vi "averager.vi"() -> ()   [LabVIEW 2015]
uses:
  <vilib>/Utility/file.llb/Write Delimited Spreadsheet (DBL).vi
  <vilib>/imath/engines/lvmath2/RunTimeEngine/Managers/WorkSpace/UID Generator.vi
  <vilib>/imath/engines/lvmath2/RunTimeEngine/BuiltInFunctions/length/NIMS_length(GV).vi
  <instcachedir>/0/NIMS_length(GV)_08A3D13377FD4E4B96F5795FBF3698FA.lvgen/NIMS_length(GV)_08A3D13377FD4E4B96F5795FBF3698FA_000.vi
  <vilib>/imath/engines/lvmath2/RunTimeEngine/RangeToken/NIMS_Range_R2 - Integer.vi
  <instcachedir>/0/NIMS_Range_R2 - Integer_396D5D4FB869421F9245109A0975AD54.lvgen/NIMS_Range_R2 - Integer_396D5D4FB869421F9245109A0975AD54_000.vi
  <vilib>/imath/engines/lvmath2/RunTimeEngine/CommandStatement/MC_CommandStatement_break.vi
  <vilib>/imath/engines/lvmath2/RunTimeEngine/VariableToken/NIMS_VariableToken_CondDefinedDefinedByReplace.vi
  <instcachedir>/0/NIMS_VariableToken_CondDefinedDefinedByReplace_D162CFFC24174562A9FEA619A91E1A56.lvgen/NIMS_VariableToken_CondDefinedDefinedByReplace_D162CFFC24174562A9FEA619A91E1A56_002.vi
  <vilib>/imath/engines/lvmath2/RunTimeEngine/IndexRead/NIMS V(S).vi
  <instcachedir>/0/NIMS V(S)_0488751826AF41519A22953C041130DC.lvgen/NIMS V(S)_0488751826AF41519A22953C041130DC_000.vi
  <vilib>/imath/engines/lvmath2/RunTimeEngine/IndexReplace/NIMS V(S)=S.vi
  <instcachedir>/0/NIMS V(S)=S_9916D32195284AEB9D40BA9A64F3B0C5.lvgen/NIMS V(S)=S_9916D32195284AEB9D40BA9A64F3B0C5_000.vi
  <vilib>/imath/engines/lvmath2/RunTimeEngine/RunTimeType/NIMS_RunTimeType_From StrictType (excl LVString).vi
  <instcachedir>/0/NIMS_RunTimeType_From StrictType (excl LVString)_EB1C38A9BC5048DA9ABDA8F781E54D21.lvgen/NIMS_RunTimeType_From StrictType (excl LVString)_EB1C38A9BC5048DA9ABDA8F781E54D21_000.vi
  <vilib>/imath/engines/lvmath2/RunTimeEngine/ErrorHandling/NIMS_Create Error From Enums.vi
  <vilib>/imath/engines/lvmath2/RunTimeEngine/LocalVariableDefStatement/MC_LocalVariableDefStatement_Display.vi
  <vilib>/imath/engines/lvmath2/RunTimeEngine/VariableToken/NIMS_VariableToken_CondDefined.vi
  <instcachedir>/0/NIMS_VariableToken_CondDefined_FE30D0A1BFB24F098D41DEBABFE96BE1.lvgen/NIMS_VariableToken_CondDefined_FE30D0A1BFB24F098D41DEBABFE96BE1_003.vi
  <vilib>/imath/engines/lvmath2/RunTimeEngine/BuiltInFunctions/sum/NIMS_sum(GV).vi
  <instcachedir>/0/NIMS_sum(GV)_67F5EC36BC034E54A6BEC5B0673C00E5.lvgen/NIMS_sum(GV)_67F5EC36BC034E54A6BEC5B0673C00E5_000.vi
  <vilib>/imath/engines/lvmath2/RunTimeEngine/Managers/SymbolTable/Clear UID.vi
  <vilib>/imath/engines/lvmath2/RunTimeEngine/NodeEndStatement/NIMS_NodeEndStatement_Output.vi
  <instcachedir>/0/NIMS_NodeEndStatement_Output_53EC0D466D134D7ABD903AC30B43404B.lvgen/NIMS_NodeEndStatement_Output_53EC0D466D134D7ABD903AC30B43404B_001.vi
  <vilib>/imath/engines/lvmath2/RunTimeEngine/ErrorHandling/NIMS_Finalize Error.vi
  <vilib>/imath/engines/lvmath2/RunTimeEngine/Managers/SymbolTable/NIMS_WorkSpace.lvlib
panel:
  in  "R2":dbl
  out "Average Resistance":dbl
  in  "Path":path
  out "data 5":dbl
  out "data 4":dbl
  out "data 3":dbl
  out "data 2":dbl
  out "data":dbl
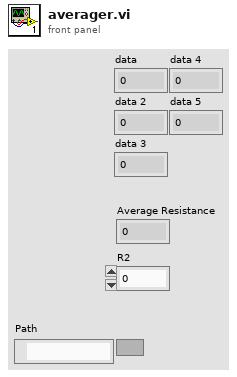
[diagram p1: front panel]
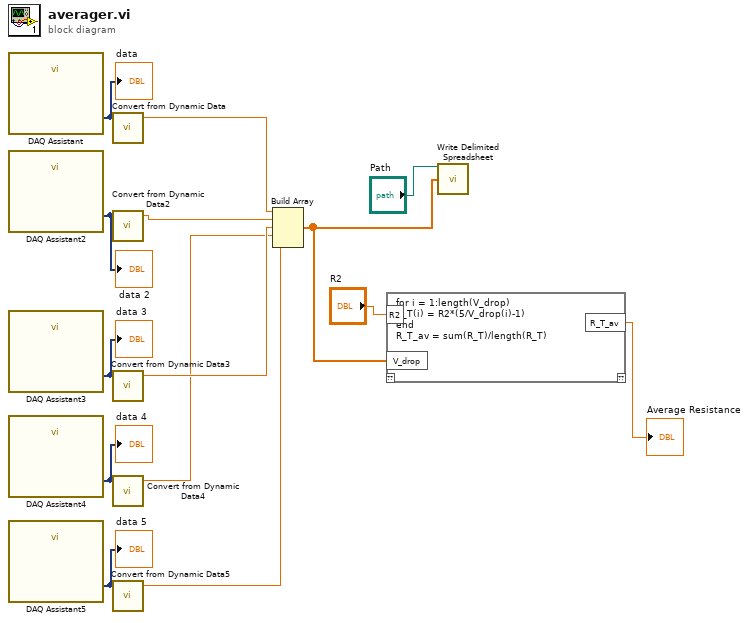
[diagram p0: block diagram]
diagram:
  n1 = call "DAQ Assistant"() -> ("data"=w14:dynamicdata)  [unwired: 17 in, 2 out]
  "data" <- w14
  n2 = call "DAQ Assistant2"() -> ("data"=w10:dynamicdata)  [unwired: 17 in, 2 out]
  "data 2" <- w10
  n3 = call "DAQ Assistant3"() -> ("data"=w11:dynamicdata)  [unwired: 17 in, 2 out]
  "data 3" <- w11
  n4 = call "DAQ Assistant4"() -> ("data"=w12:dynamicdata)  [unwired: 17 in, 2 out]
  "data 4" <- w12
  n5 = call "DAQ Assistant5"() -> ("data"=w13:dynamicdata)  [unwired: 17 in, 2 out]
  "data 5" <- w13
  n6 = call "Convert from Dynamic Data"("Dynamic Data Type"=w14) -> ("Scalar"=w9:dbl)  [unwired: 3 in]
  n7 = call "Convert from Dynamic Data2"("Dynamic Data Type"=w10) -> ("Scalar"=w8:dbl)  [unwired: 3 in]
  n8 = call "Convert from Dynamic Data3"("Dynamic Data Type"=w11) -> ("Scalar"=w7:dbl)  [unwired: 3 in]
  n9 = call "Convert from Dynamic Data4"("Dynamic Data Type"=w12) -> ("Scalar"=w6:dbl)  [unwired: 3 in]
  n10 = call "Convert from Dynamic Data5"("Dynamic Data Type"=w13) -> ("Scalar"=w5:dbl)  [unwired: 3 in]
  n11 = Build Array(w9, w8, w7, w6, w5) -> (w2:dbl[])
  n12 = mathscript code="for i = 1:length(V_drop)\nR_T(i) = R2*(5/V_drop(i)-1)\nend\nR_T_av = sum(R_T)/length(R_T)"("R2"="R2", "V_drop"=w2) -> ("R_T_av"=→"Average Resistance":dbl)  [unwired: 1 in, 1 out]
  n13 = call-poly <vilib>:"Write Delimited Spreadsheet.vi"("file path (dialog if empty)"="Path", "1D data"=w2) -> ()  [unwired: 12 in, 2 out]
